vi "Open Form.vi"(6 "Custom Form Model Config":refnum<class "Form Model Configuration.lvclass">, 7 "Name":string, 8 "error in (no error)":errorcluster, 9 "Sub Panel Refnum":refnum<vi>, 10 "Form":refnum<class "Panel Form Controller.lvclass">, 11 "Form Server Wrapper in":refnum<class "Form Server Wrapper.lvclass">) -> (0 "error out":errorcluster, 3 "Form Server Wrapper out":refnum<class "Form Server Wrapper.lvclass">)   [LabVIEW 2020, in "Form Server.lvlib" / "Form Server Wrapper.lvclass"]
uses:
  Form Server Wrapper.lvclass
  Form Model/Form Configuration/Form Model Configuration.lvclass
  Form Controller/Panel Form Controller.lvclass
  Autoclose manager/Form ID.ctl
  Form Server Wrapper.lvclass/Form Server Wrapper.ctl
  Form Server Messages Messages/Open Form Msg/Open Form Msg.lvclass/Open Form Msg.ctl
  <vilib>/ActorFramework/Message Enqueuer/Message Enqueuer.lvclass/Message Enqueuer.ctl
  <vilib>/ActorFramework/Message Enqueuer/Enqueue.vi
  Database OOP/Table Libraries/Basic Table/Configuration/Table Configuration Adv Schema DB/Table Configuration Adv Schema DB.lvclass
  C:/Users/User/Desktop/Raman Program/Database OOP/source/Database OOP/Table Libraries/Table Configuration Interface/Table Configuration Interface.lvclass
  Form from Table Configuration/Form from Table Configuration.lvclass
  C:/Users/User/Desktop/Raman Program/Database OOP/source/Forms AF/Controller Configuration/Panel Form Controller Configuration.lvclass
  <vilib>/MGI/Panel Manager/Panel/Panel/Window/Window.lvclass
  C:/Program Files (x86)/National Instruments/LabVIEW 2020/vi.lib/MGI/Panel Manager/Panel/Panel/Panel.lvclass
  <vilib>/MGI/Panel Manager/Panel/Panel/Subpanel/Subpanel.lvclass
  Form Model/Model Panel Logic/Model Panel Logic Nested Window.lvclass
  C:/Users/User/Desktop/Raman Program/Database OOP/source/Forms AF/Model Panel Logic/Model Panel Logic.lvclass
  Form Server Messages Messages/Open Form Msg/Open Form Msg.lvclass
  C:/Program Files (x86)/National Instruments/LabVIEW 2020/vi.lib/ActorFramework/Message/Message.lvclass
  Database OOP/Table Libraries/Basic Table/Configuration/Table Configuration Adv Schema DB/Table Constructor Adv Schema DB.vi
  Form from Table Configuration/Constructor by Table Config.vi
  <vilib>/MGI/Panel Manager/Panel/Panel/Window/Window.vi
  <vilib>/MGI/Panel Manager/Panel/Panel/Subpanel/Subpanel.vi
  <vilib>/ActorFramework/Message Priority Queue/Priority Enqueue.vi
  <vilib>/MGI/Panel Manager/Panel/Panel.lvlib
  Panel Form Controller.lvlib
  Database OOP/Table Libraries/Table.lvlib
  Form Server Interfaces.lvlib
  C:/Users/User/Desktop/Raman Program/Database OOP/source/Database OOP/Table Libraries/Basic Table/Configuration/Table Configuration Class/Table Configuration.lvclass
  C:/Users/User/Desktop/Raman Program/Database OOP/source/Database OOP/Table Libraries/Basic Table/Configuration/Table Configuration Adv Schema DB/Table Configuration Adv Schema DB.lvclass
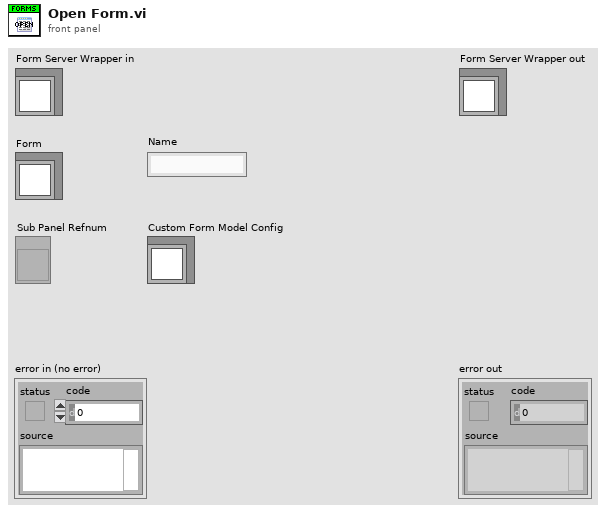
[diagram p1: front panel]
types:
  T1 = typedef "Form Server Interfaces.lvlib/Form ID.ctl" = cluster{"Name":string, "Panel type":string}
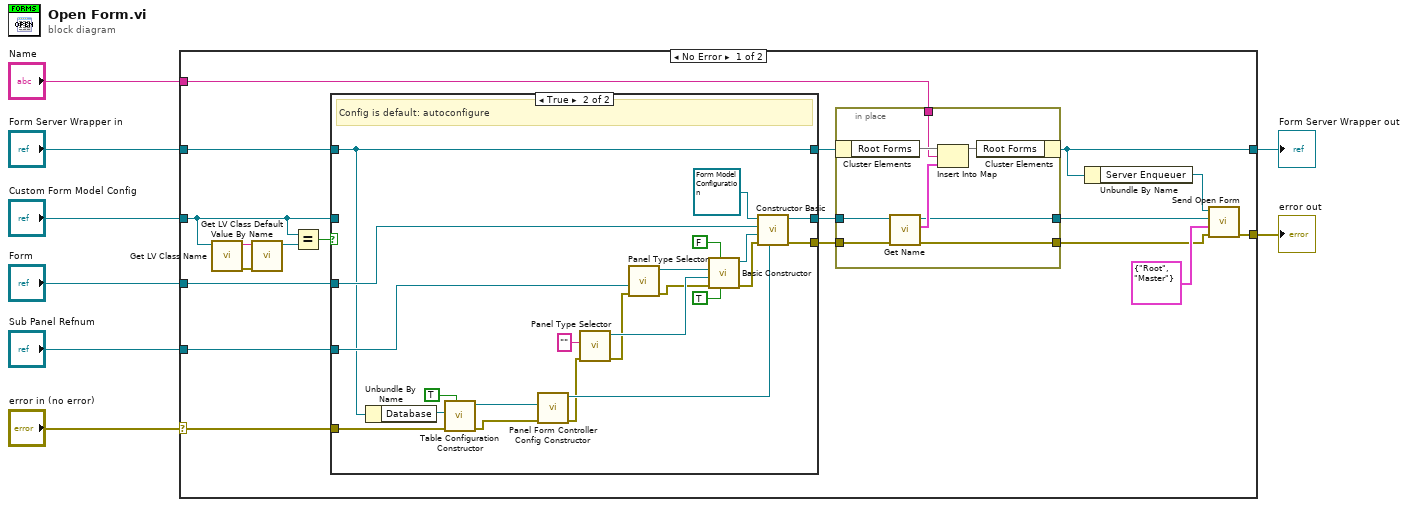
[diagram p0: block diagram]
diagram:
  n1 = case shown="No Error" "error in (no error)" {
    selector: "error in (no error)" -> [w20 w62]
    tunnel: [w9 w62] -> w7
    tunnel: [w10 w61] -> w5
    tunnel: "Form Server Wrapper in" -> [w23 w61]
    tunnel: "Custom Form Model Config" -> [w19 _]
    tunnel: "Form" -> [w22 _]
    tunnel: "Sub Panel Refnum" -> [w21 _]
    tunnel: "Name" -> [w13 _]
    frame No Error {
      n2 = call <vilib>:"Get LV Class Name.vi"("object"=w19) -> ("error out"=w27:errorcluster, "class name"=w26:string)  [unwired: 9 in]
      n3 = call <vilib>:"Get LV Class Default Value By Name.vi"("error in (no error)"=w27, "class name"=w26) -> ("object"=w25:refnum<class>)  [unwired: 8 in, 1 out]
      n4 = Equal?(x=w19, y=w25) -> (x = y?=w24:bool)
      n5 = case shown="True" w24 {
        tunnel: w23 -> [w36 w41]
        tunnel: w22 -> [_ w43]
        tunnel: w21 -> [_ w44]
        tunnel: w20 -> [w37 w42]
        tunnel: [w36 w41] -> w16
        tunnel: [w38 w40] -> w15
        tunnel: [w37 w39] -> w14
        tunnel: w19 -> [w38 _]
        frame False {
          # "Already Configured"
        }
        frame True {
          # "Config is default: autoconfigure"
          n6 = Unbundle By Name(w41) -> ("Database"=w51:refnum<class "Database Adv Schema.lvclass">)
          n7 = call-poly "Table Configuration Constructor.vi"("Defer Constructor (F)"=TRUE, "error in (no error)"=w42, "Database"=w51) -> ("error out"=w49:errorcluster, "Table Configuration Adv Schema DB out"=w52:refnum<class "Table Configuration Adv Schema DB.lvclass">)  [unwired: 7 in]
          n8 = call-poly "Panel Form Controller Config Constructor.vi"("error in (no error)"=w49, "Table Configuration"=w52) -> ("error out"=w48:errorcluster, "Form from Table Configuration out"=w50:refnum<class "Form from Table Configuration.lvclass">)  [unwired: 8 in]
          n9 = call-poly <vilib>:"Panel Type Selector.vi"("error in (no error)"=w48, "Default Title"="") -> ("error out"=w47:errorcluster, "Window out"=w58:refnum<class "Window.lvclass">)  [unwired: 8 in]
          n10 = call-poly <vilib>:"Panel Type Selector.vi"("Error In"=w47, "Sub Panel"=w44) -> ("Error Out"=w46:errorcluster, "Subpanel Out"=w57:refnum<class "Subpanel.lvclass">)  [unwired: 8 in]
          n11 = call "Basic Constructor.vi"("Nested panels for additional? (T)"=TRUE, "Nested panels for root? (F)"=FALSE, "error in (no error)"=w46, "Additional Panels (window)"=w58, "Root Panel"=w57) -> ("error out"=w45:errorcluster, "Model Panel Logic out"=w54:refnum<class "Model Panel Logic Nested Window.lvclass">)  [unwired: 5 in]
          n12 = call "Constructor Basic.vi"("Controller Config"=w50, "error in (no error)"=w45, "Panel Logic"=w54, "Panel Form Controller"=w43, "Form Model Configuration in"=refnum<class "Form Model Configuration.lvclass"> refnum) -> ("error out"=w39:errorcluster, "Form Model Configuration out"=w40:refnum<class "Form Model Configuration.lvclass">)  [unwired: 5 in]
        }
      }
      n13 = in-place {
        in-place-border: w15 -> [w35]
        in-place-border: w14 -> [w34]
        in-place-border: w13 -> [w30]
        in-place-border: [w29] -> w12
        in-place-border: [w28] -> w11
        n14 = in-place-cluster #1(w16) -> ("Root Forms"=w33:map{string, T1})
        n15 = call-dynamic "Get Name.vi"("error in (no error)"=w34, "Form Configuration in"=w35) -> ("error out"=w28:errorcluster, "Form ID"=w31:T1, "Form Configuration out"=w29:refnum<class "Form Model Configuration.lvclass">)  [unwired: 7 in]
        n16 = Insert Into Map(map in=w33, key=w30, value=w31) -> (map out=w32:map{string, T1})  [unwired: 2 out]
        n17 = in-place-cluster #1("Root Forms"=w32) -> (w10:refnum<class "Form Server Wrapper.lvclass">)
      }
      n18 = Unbundle By Name(w10) -> ("Server Enqueuer"=w17:refnum<class "Message Enqueuer.lvclass">)
      n19 = call "Send Open Form.vi"("error in (no error)"=w11, "Caller Name"=T1 {"Name"="Root", "Panel type"="Master"}, "Form Config"=w12, "Message Enqueuer"=w17) -> ("error out"=w9:errorcluster)  [unwired: 6 in, 1 out]
    }
    frame Error {
    }
  }
  "error out" <- w7
  "Form Server Wrapper out" <- w5
